vi "β吸收.vi"() -> ()   [LabVIEW 2014]
panel:
  in  "单道1道宽/mV":u16=3000
  in  "单道1阈值/mV":i32=100
  out "电压表":u32(knob) scale=0.0..500.0
  in  "runtime(秒)":u16=10
  in  "选项卡控件_实验步骤":enum32{"选项卡 1", "选项卡 2"}(tab)
  in  "按钮_提示":bool caption="提示"
  out "电压/V":u32 max=490 step=10
  out "已用时间/s":i32
  out "停止":bool
  in  "按钮_停止测量":bool
  out "计数":i32
  out "放射源":bool
  in  "按钮_放射源":bool
  in  "铝片个数":i32 min=0 max=18 step=1
  in  "按钮_放置铝片":bool
  in  "按钮_测量":bool
  in  "数组 2":dbl[](array[numeric])
  in  "数组":u32[](array[numeric])
  in  "按钮_电压设置":bool
  in  "电压":u32 max=490 step=10
  out "退出":bool
  in  "按钮_退出":bool
  # "实验：β射线吸收"
  # "实验原理"
  # "实"
  # "单道"
  # "高压"
  # "G-M计数器"
  # "验"
  # "仪"
  # "操作面板"
  # "器"
  # "定标"
  # "电压/V"
  # "放射源"
  # "实验内容"
  # "计数"
  # "已用时间/s"
  # "铝片个数"
  # "设定时间/s"
  # "1.连接好仪器。放置放射源，测量G-M计数管的坪\n曲线，确定其工作电压。从260V开始找阈电压V0,找到\n后以10V为步长测坪曲线,测15个数据点,每点30s。\n      2.计算每片铝吸收片的质量厚度。\n      3.测量铝片对Beta射线的吸收曲线。至少测18片铝\n片。铝片质量厚度<200mg/cm2时,要求统计误差<\n2%,质量厚度200~600mg/cm2时,统计误差小于3%,质\n量厚度>600mg/cm2时,统计误差<4%。\n      4.取出放射源，其它条件不变，测量本底5分钟。"
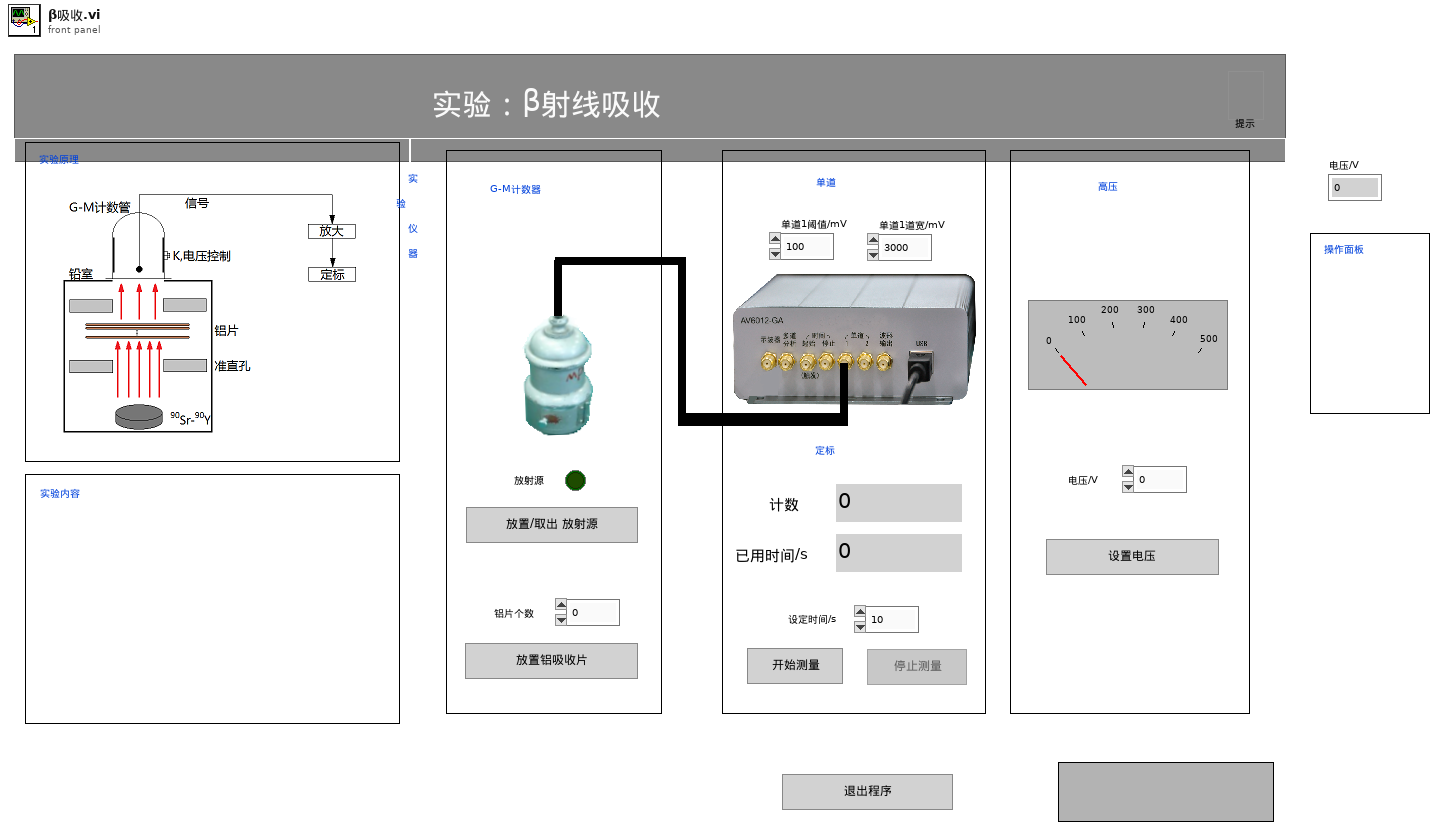
[diagram p1: front panel]
types:
  T1 = enum8{"Enabled", "Disabled", "Disabled and Grayed Out"}
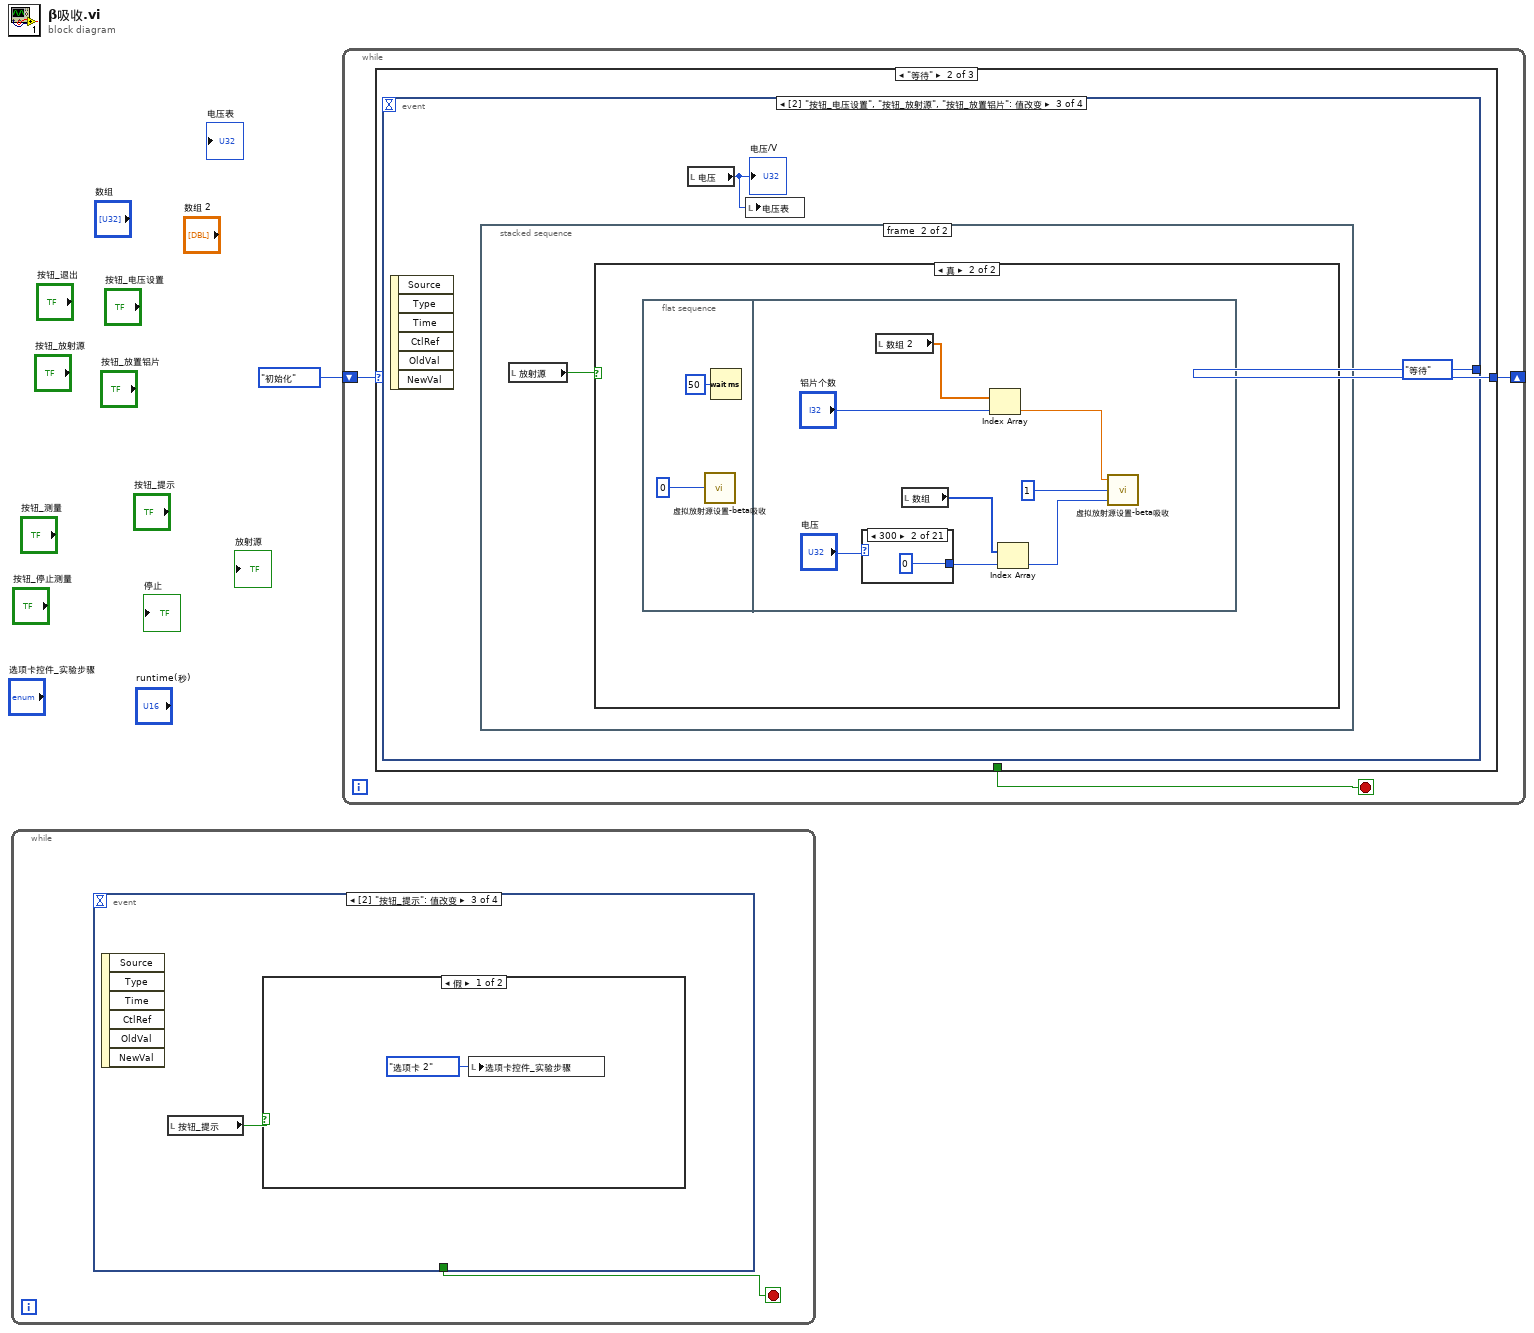
[diagram p0: block diagram]
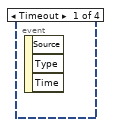
[diagram p2: hidden frame]
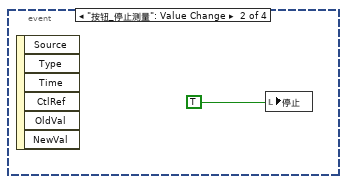
[diagram p3: hidden frame]
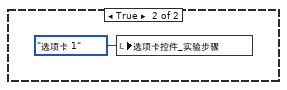
[diagram p4: hidden frame]
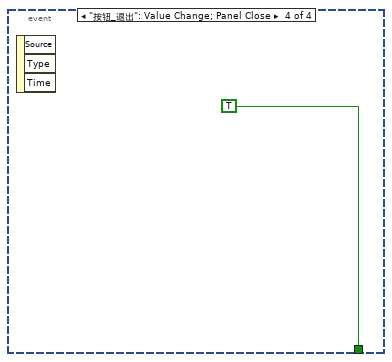
[diagram p5: hidden frame]
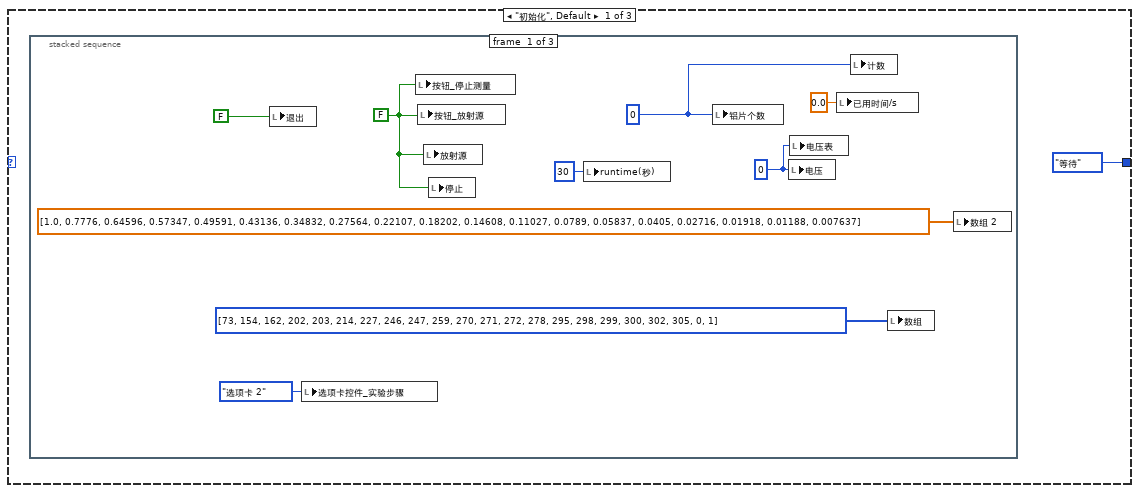
[diagram p6: hidden frame]
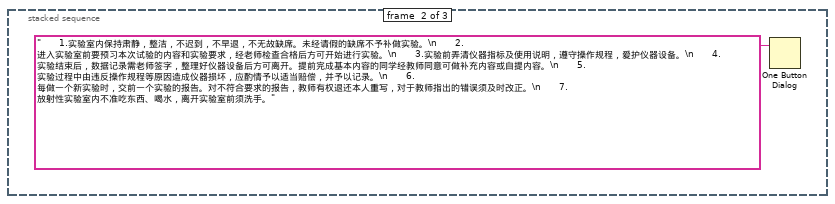
[diagram p7: hidden frame]
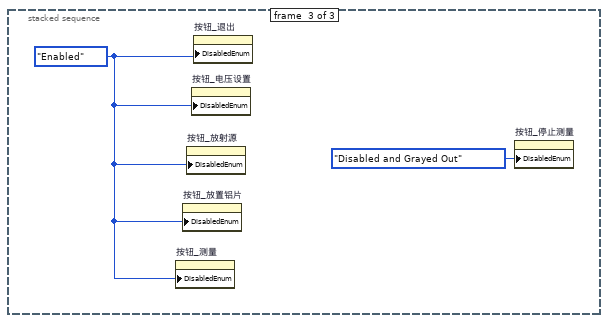
[diagram p8: hidden frame]
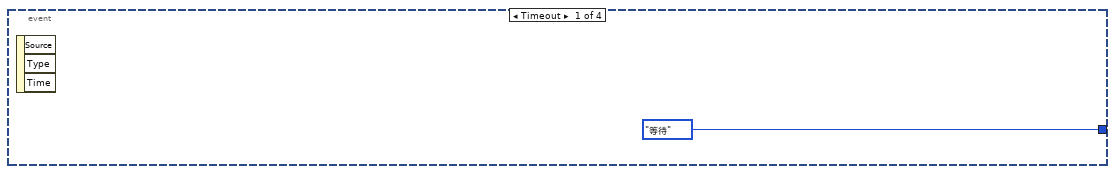
[diagram p9: hidden frame]
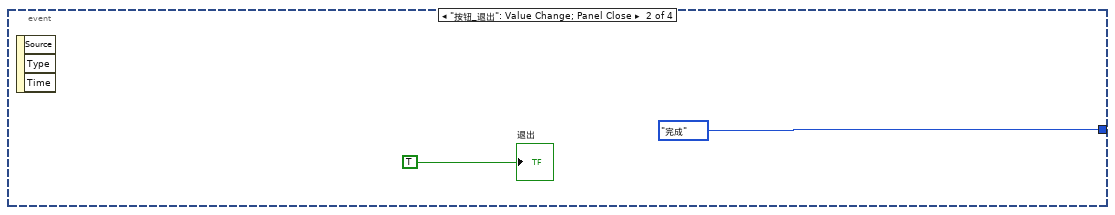
[diagram p10: hidden frame]
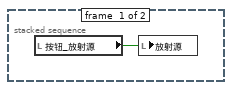
[diagram p11: hidden frame]
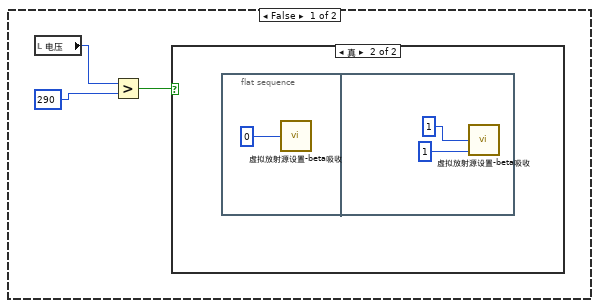
[diagram p12: hidden frame]
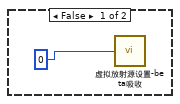
[diagram p13: hidden frame]
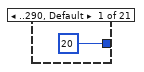
[diagram p14: hidden frame]
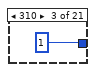
[diagram p15: hidden frame]
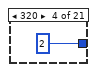
[diagram p16: hidden frame]
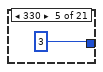
[diagram p17: hidden frame]
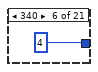
[diagram p18: hidden frame]
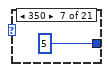
[diagram p19: hidden frame]
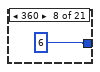
[diagram p20: hidden frame]
diagram:
  n1 = while {
    stop <- w2 stop-if-true
    n2 = event shown="[2] \"按钮_提示\": 值改变" {
      selector: _ -> [_ _ _ _]
      dyn-events: _ -> [_ _ _ _]
      timeout: _ -> [_ _ _ _]
      tunnel: [_ _ _ TRUE] -> w2
      event Timeout {
        n3 = event-data() -> ()  [unwired: 1 in, 3 out]
      }
      event "按钮_停止测量": Value Change {
        n4 = event-data() -> ()  [unwired: 1 in, 6 out]
        n5 = local write "停止"(TRUE) -> ()
      }
      event "按钮_提示": Value Change {
        n6 = event-data() -> ()  [unwired: 1 in, 6 out]
        n7 = local read "按钮_提示"() -> (w4:bool)
        n8 = case shown="假" w4 {
          frame False {
            n9 = local write "选项卡控件_实验步骤"(enum32{"选项卡 1", "选项卡 2"}."选项卡 2" ("选项卡控件_实验步骤")) -> ()
          }
          frame True {
            n10 = local write "选项卡控件_实验步骤"(enum32{"选项卡 1", "选项卡 2"}."选项卡 1" ("选项卡控件_实验步骤")) -> ()
          }
        }
      }
      event "按钮_退出": Value Change; Panel Close {
        n11 = event-data() -> ()  [unwired: 1 in, 3 out]
      }
    }
  }
  n12 = while {
    shift-right: [w8] -> _
    shift-left: enum16{"初始化", "等待", "完成"}."初始化" -> [w10]
    stop <- w9 stop-if-true
    n13 = case shown="\"等待\"" w10 {
      tunnel: [_ _ TRUE] -> w9
      tunnel: [enum16{"初始化", "等待", "完成"}."等待" w24 enum16{"初始化", "等待", "完成"}."完成"] -> w8
      frame "初始化", Default {
        n14 = stacked-sequence {
          frame #0 {
            w12 = u32 0 ("电压")
            w17 = 0
            w13 = FALSE
            n15 = local write "退出"(FALSE) -> ()
            n16 = local write "选项卡控件_实验步骤"(enum32{"选项卡 1", "选项卡 2"}."选项卡 2" ("选项卡控件_实验步骤")) -> ()
            n17 = local write "按钮_停止测量"(w13) -> ()
            n18 = local write "按钮_放射源"(w13) -> ()
            n19 = local write "放射源"(w13) -> ()
            n20 = local write "停止"(w13) -> ()
            n21 = local write "runtime(秒)"(u16 30 ("runtime(秒)")) -> ()
            n22 = local write "铝片个数"(w17) -> ()
            n23 = local write "电压"(w12) -> ()
            n24 = local write "电压表"(w12) -> ()
            n25 = local write "已用时间/s"(0.0) -> ()
            n26 = local write "计数"(w17) -> ()
            n27 = local write "数组"(u32[] [73, 154, 162, 202, 203, 214, 227, 246, 247, 259, 270, 271, 272, 278, 295, 298, 299, 300, 302, 305, 0, 1]) -> ()
            n28 = local write "数组 2"(dbl[] [1.0, 0.7776, 0.64596, 0.57347, 0.49591, 0.43136, 0.34832, 0.27564, 0.22107, 0.18202, 0.14608, 0.11027, 0.0789, 0.05837, 0.0405, 0.02716, 0.01918, 0.01188, 0.007637]) -> ()
          }
          frame #1 {
            n29 = One Button Dialog(message="      1.实验室内保持肃静，整洁，不迟到，不早退，不无故缺席。未经请假的缺席不予补做实验。\n      2.进入实验室前要预习本次试验的内容和实验要求，经老师检查合格后方可开始进行实验。\n      3.实验前弄清仪器指标及使用说明，遵守操作规程，爱护仪器设备。\n      4.实验结束后，数据记录需老师签字，整理好仪器设备后方可离开。提前完成基本内容的同学经教师同意可做补充内容或自提内容。\n      5.实验过程中由违反操作规程等原因造成仪器损坏，应酌情予以适当赔偿，并予以记录。\n      6.每做一个新实验时，交前一个实验的报告。对不符合要求的报告，教师有权退还本人重写，对于教师指出的错误须及时改正。\n      7.放射性实验室内不准吃东西、喝水，离开实验室前须洗手。" ("消息")) -> ()  [unwired: 1 in, 1 out]
          }
          frame #2 {
            w23 = T1."Enabled" ("禁用")
            n30 = property on="按钮_测量" class="Bool (严格)"("DisabledEnum"=w23) -> ()  [unwired: 2 in, 2 out]
            n31 = property on="按钮_放置铝片" class="Bool (严格)"("DisabledEnum"=w23) -> ()  [unwired: 2 in, 2 out]
            n32 = property on="按钮_放射源" class="Bool (严格)"("DisabledEnum"=w23) -> ()  [unwired: 2 in, 2 out]
            n33 = property on="按钮_电压设置" class="Bool (严格)"("DisabledEnum"=w23) -> ()  [unwired: 2 in, 2 out]
            n34 = property on="按钮_退出" class="Bool (严格)"("DisabledEnum"=w23) -> ()  [unwired: 2 in, 2 out]
            n35 = property on="按钮_停止测量" class="Bool (严格)"("DisabledEnum"=T1."Disabled and Grayed Out" ("禁用")) -> ()  [unwired: 2 in, 2 out]
          }
        }
      }
      frame "等待" {
        n36 = event shown="[2] \"按钮_电压设置\", \"按钮_放射源\", \"按钮_放置铝片\": 值改变" {
          selector: _ -> [_ _ _ _]
          dyn-events: _ -> [_ _ _ _]
          timeout: _ -> [_ _ _ _]
          tunnel: [enum16{"初始化", "等待", "完成"}."等待" enum16{"初始化", "等待", "完成"}."完成" enum16{"初始化", "等待", "完成"}."等待" enum16{"初始化", "等待", "完成"}."等待"] -> w24
          event Timeout {
            n37 = event-data() -> ()  [unwired: 1 in, 3 out]
          }
          event "按钮_退出": Value Change; Panel Close {
            n38 = event-data() -> ()  [unwired: 1 in, 3 out]
            "退出" <- TRUE
          }
          event "按钮_电压设置", "按钮_放射源", "按钮_放置铝片": Value Change {
            n39 = event-data() -> ()  [unwired: 1 in, 6 out]
            n40 = stacked-sequence {
              frame #0 {
                n41 = local read "按钮_放射源"() -> (w30:bool)
                n42 = local write "放射源"(w30) -> ()
              }
              frame #1 {
                n43 = local read "放射源"() -> (w31:bool)
                n44 = case shown="真" w31 {
                  frame False {
                    n45 = local read "电压"() -> (w34:u32)
                    n46 = Greater?(x=w34, y=290) -> (0:w32:bool)
                    n47 = case shown="真" w32 {
                      frame False {
                        n48 = call "虚拟放射源设置-beta吸收.vi"("仪器使能"=0) -> ()  [unwired: 2 in]
                      }
                      frame True {
                        n49 = flat-sequence {
                          frame #0 {
                            n50 = call "虚拟放射源设置-beta吸收.vi"("仪器使能"=0) -> ()  [unwired: 2 in]
                          }
                          frame #1 {
                            n51 = call "虚拟放射源设置-beta吸收.vi"("计数率"=1, "仪器使能"=1) -> ()  [unwired: 1 in]
                          }
                        }
                      }
                    }
                  }
                  frame True {
                    n52 = flat-sequence {
                      frame #0 {
                        n53 = call "虚拟放射源设置-beta吸收.vi"("仪器使能"=0) -> ()  [unwired: 2 in]
                        n54 = Wait (ms)(milliseconds to wait=50) -> ()  [unwired: 1 out]
                      }
                      frame #1 {
                        n55 = case shown="300" "电压" {
                          tunnel: [20 0 1 2 3 4 5 6 7 8 9 10 11 12 13 14 15 16 17 18 19] -> w48
                          frame ..290, Default {
                          }
                          frame 300 {
                          }
                          frame 310 {
                          }
                          frame 320 {
                          }
                          frame 330 {
                          }
                          frame 340 {
                          }
                          frame 350 {
                          }
                          frame 360 {
                          }
                          frame 370 {
                          }
                          frame 380 {
                          }
                          frame 390 {
                          }
                          frame 400 {
                          }
                          frame 410 {
                          }
                          frame 420 {
                          }
                          frame 430 {
                          }
                          frame 440 {
                          }
                          frame 450 {
                          }
                          frame 460 {
                          }
                          frame 470 {
                          }
                          frame 480 {
                          }
                          frame 490 {
                          }
                        }
                        n56 = local read "数组 2"() -> (w42:dbl[])
                        n57 = local read "数组"() -> (w47:u32[])
                        n58 = Index Array(array=w42, index="铝片个数") -> (element=w41:dbl)
                        n59 = Index Array(array=w47, index=w48) -> (element=w45:u32)
                        n60 = call "虚拟放射源设置-beta吸收.vi"("计数率"=w45, "仪器使能"=1, "衰减系数"=w41) -> ()
                      }
                    }
                  }
                }
              }
            }
            n61 = local read "电压"() -> (w28:u32)
            "电压/V" <- w28
            n62 = local write "电压表"(w28) -> ()
          }
          event "按钮_测量": Value Change {
            n63 = event-data() -> ()  [unwired: 1 in, 6 out]
            n64 = stacked-sequence {
              frame #0 {
                w75 = T1."Disabled and Grayed Out" ("禁用")
                n65 = property on="按钮_放置铝片" class="Bool (严格)"("DisabledEnum"=w75) -> ()  [unwired: 2 in, 2 out]
                n66 = property on="按钮_放射源" class="Bool (严格)"("DisabledEnum"=w75) -> ()  [unwired: 2 in, 2 out]
                n67 = property on="按钮_电压设置" class="Bool (严格)"("DisabledEnum"=w75) -> ()  [unwired: 2 in, 2 out]
                n68 = property on="按钮_退出" class="Bool (严格)"("DisabledEnum"=w75) -> ()  [unwired: 2 in, 2 out]
                n69 = property on="按钮_测量" class="Bool (严格)"("DisabledEnum"=w75) -> ()  [unwired: 2 in, 2 out]
                n70 = property on="按钮_停止测量" class="Bool (严格)"("DisabledEnum"=T1."Enabled" ("禁用")) -> ()  [unwired: 2 in, 2 out]
                n71 = call "chushihua.vi"("单道1道宽"="单道1道宽/mV", "runtime(秒)"=u16 65535, "单道1阈值"="单道1阈值/mV") -> ()
              }
              frame #1 {
                n72 = call "发送.vi"("命令(16bit)"="\u0000\n", "目标IP"="192.168.0.2") -> ()  [unwired: 1 in, 1 out]
              }
              frame #2 {
                n73 = Tick Count (ms)() -> (millisecond timer value=w78:u32)
                n74 = while {
                  tunnel: w78 -> [w86]
                  stop <- w79 stop-if-true
                  n75 = call "读取.vi"("命令"="\u0000\u000b", "帧数"=1) -> ("数组"=w89:string[])  [unwired: 1 out]
                  n76 = Tick Count (ms)() -> (millisecond timer value=w87:u32)
                  n77 = Index Array(array=w89, index=0 ("索引")) -> (element=w88:string)
                  n78 = Subtract(x=w87, y=w86) -> (x-y=w85:u32)
                  n79 = String Subset(string=w88, offset (0)=0 ("偏移量(0)"), length (rest)=4 ("长度（剩余）")) -> (substring=w94:string)
                  n80 = String To Byte Array(string=w94) -> (unsigned byte array=w93:u8[])
                  n81 = local read "runtime(秒)"() -> (w82:u16)
                  n82 = Divide(x=w85, y=1000) -> (x/y=w83:dbl)
                  "已用时间/s" <- w83
                  n83 = Decimate 1D Array(w93) -> (w95:u8[], w96:u8[], w106:u8[], w105:u8[])
                  n84 = Multiply(x=256, y=w106) -> (x*y=w101:i32[])
                  n85 = Multiply(x=1, y=w105) -> (x*y=w102:i32[])
                  n86 = Multiply(x=65536, y=w96) -> (x*y=w98:i32[])
                  n87 = Multiply(x=16777216, y=w95) -> (x*y=w97:i32[])
                  n88 = Greater Or Equal?(x=w83, y=w82) -> (x >= y?=w81:bool)
                  n89 = Compound Arithmetic op=ADD(w97, w98, w101, w102) -> (w92:i32[])
                  n90 = Index Array(array=w92, index=0 ("索引")) -> (element=→"计数":i32)
                  n91 = local read "停止"() -> (w80:bool)
                  n92 = Or(x=w80, y=w81) -> (x .or. y?=w79:bool)
                }
              }
              frame #3 {
                w112 = T1."Enabled" ("禁用")
                n93 = property on="按钮_放置铝片" class="Bool (严格)"("DisabledEnum"=w112) -> ()  [unwired: 2 in, 2 out]
                n94 = property on="按钮_放射源" class="Bool (严格)"("DisabledEnum"=w112) -> ()  [unwired: 2 in, 2 out]
                n95 = property on="按钮_电压设置" class="Bool (严格)"("DisabledEnum"=w112) -> ()  [unwired: 2 in, 2 out]
                n96 = property on="按钮_退出" class="Bool (严格)"("DisabledEnum"=w112) -> ()  [unwired: 2 in, 2 out]
                n97 = property on="按钮_测量" class="Bool (严格)"("DisabledEnum"=w112) -> ()  [unwired: 2 in, 2 out]
                n98 = property on="按钮_停止测量" class="Bool (严格)"("DisabledEnum"=T1."Disabled and Grayed Out" ("禁用")) -> ()  [unwired: 2 in, 2 out]
                n99 = local write "停止"(FALSE ("停止")) -> ()
              }
            }
          }
        }
      }
      frame "完成" {
      }
    }
  }
